vi "parse_heart_rate_sensaura.vi"(8 "error in (no error)":errorcluster, 10 "Handle table":string[][](array[string]), 11 "payload":u8[](array[numeric])) -> (0 "error out":errorcluster, 2 "RR (ms)":u16[](array[numeric]), 3 "HR (bpm)":u16)   [LabVIEW 2015]
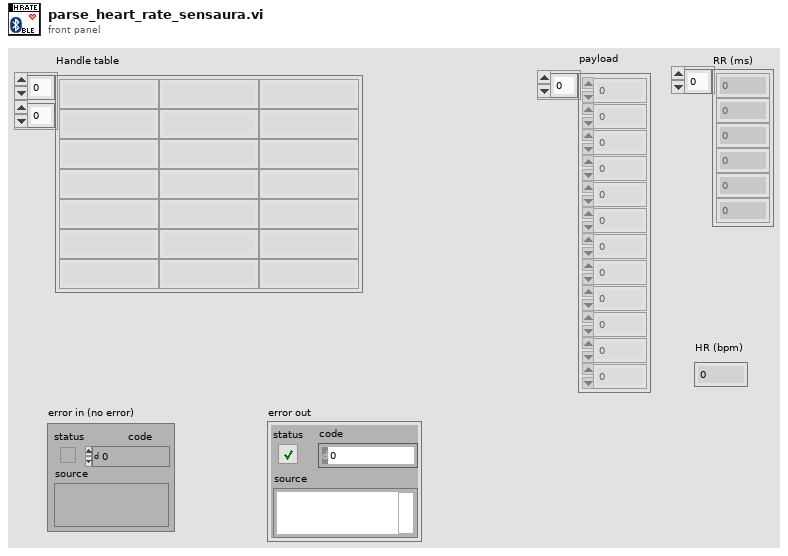
[diagram p1: front panel]
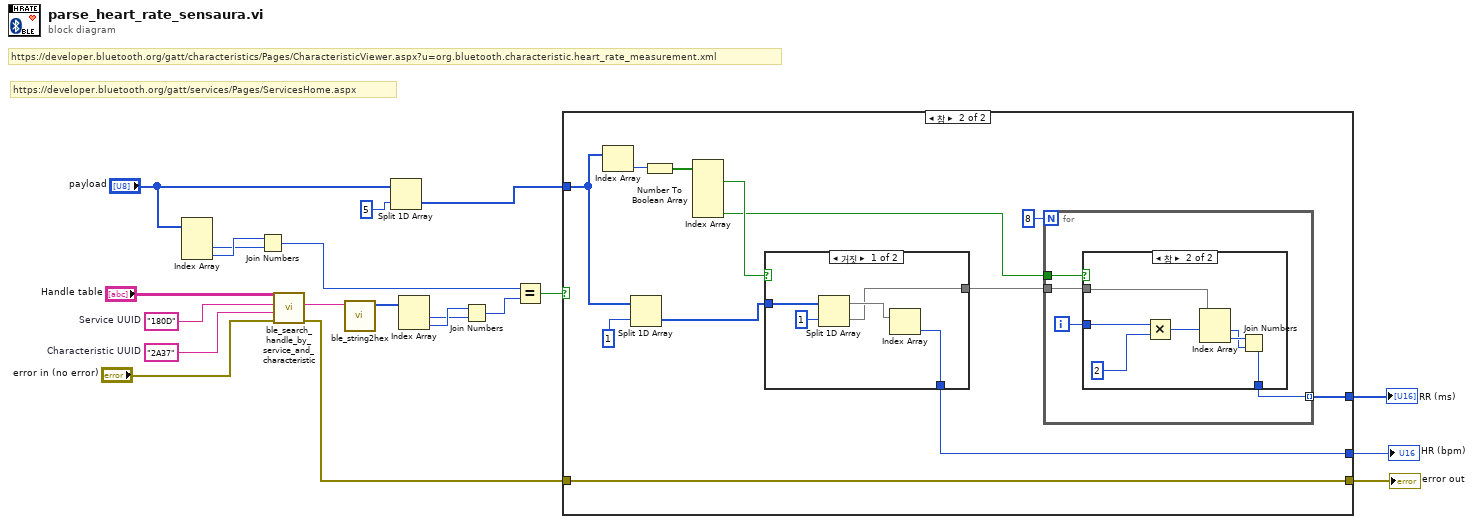
[diagram p0: block diagram]
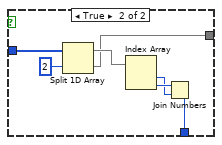
[diagram p4: hidden frame]
diagram:
  w18 = "2A37"  # Characteristic UUID
  w19 = "180D"  # Service UUID
  # "https://developer.bluetooth.org/gatt/services/Pages/ServicesHome.aspx"
  # "https://developer.bluetooth.org/gatt/characteristics/Pages/CharacteristicViewer.aspx?u=org.bluetooth.characteristic.heart_rate_measurement.xml"
  n1 = Index Array(array="payload") -> (element #2=w11:u8, element #3=w12:u8)  [unwired: 3 in, 1 out]
  n2 = Join Numbers(hi=w12, lo=w11) -> ((hi.lo)=w9:u16)
  n3 = call <vilib>:"ble_search_handle_by_service_and_characteristic.vi"("error in (no error)"="error in (no error)", "Characteristic UUID"=w18, "Service UUID"=w19, "Handle table"="Handle table") -> ("error out"=w7:errorcluster, "Handle"=w13:string)  [unwired: 6 in]
  n4 = call <vilib>:"ble_string2hex.vi"("HEX string IN"=w13) -> ("Byte Array IN (index0 LS byte)"=w16:u8[])  [unwired: 10 in]
  n5 = Split 1D Array(array="payload", index=5) -> (second subarray=w3:u8[])  [unwired: 1 out]
  n6 = Index Array(array=w16) -> (element #1=w14:u8, element #2=w15:u8)  [unwired: 2 in]
  n7 = Join Numbers(hi=w15, lo=w14) -> ((hi.lo)=w10:u16)
  n8 = Equal?(x=w9, y=w10) -> (x = y?=w8:bool)
  n9 = case shown="참" w8 {
    tunnel: w3 -> [_ w26]
    tunnel: w7 -> [w21 w33]
    tunnel: [w21 w33] -> w6
    tunnel: [_ w29] -> w2
    tunnel: [_ w27] -> w1
    frame False {
    }
    frame True {
      n10 = Index Array(array=w26) -> (element=w32:u8)  [unwired: 1 in]
      n11 = Split 1D Array(array=w26, index=1) -> (second subarray=w25:u8[])  [unwired: 1 out]
      n12 = Number To Boolean Array(number=w32) -> (Boolean array=w31:bool[])
      n13 = Index Array(array=w31) -> (element #1=w30:bool, element #5=w28:bool)  [unwired: 5 in, 3 out]
      n14 = case shown="거짓" w30 {
        tunnel: w25 -> [w47 w56]
        tunnel: [w46 w51] -> w29
        tunnel: [w45 w50] -> w23
        frame False {
          n15 = Split 1D Array(array=w47, index=1) -> (first subarray=w48:u8[], second subarray=w45:u8[])
          n16 = Index Array(array=w48) -> (element=w46:u8)  [unwired: 1 in]
        }
        frame True {
          n17 = Split 1D Array(array=w56, index=2) -> (first subarray=w54:u8[], second subarray=w50:u8[])
          n18 = Index Array(array=w54) -> (element #1=w52:u8, element #2=w53:u8)  [unwired: 2 in]
          n19 = Join Numbers(hi=w53, lo=w52) -> ((hi.lo)=w51:u16)
        }
      }
      n20 = for {
        N: 8 -> [_]
        tunnel: w28 -> [w37]
        tunnel: [w36] -> w27 mode=indexing
        tunnel: w23 -> [w35]
        i -> [w34]
        n21 = case shown="참" w37 {
          tunnel: w35 -> [_ w41]
          tunnel: [_ w42] -> w36
          tunnel: w34 -> [_ w38]
          frame False {
          }
          frame True {
            n22 = Multiply(x=w38, y=2 ("index")) -> (x*y=w40:i32)
            n23 = Index Array(array=w41, index #1=w40) -> (element #1=w43:u8, element #2=w44:u8)  [unwired: 1 in]
            n24 = Join Numbers(hi=w44, lo=w43) -> ((hi.lo)=w42:u16)
          }
        }
      }
    }
  }
  "error out" <- w6
  "HR (bpm)" <- w2
  "RR (ms)" <- w1
